vi "newRobotsLifeTime.vi"(7 "Life Time":dbl=2.0, 8 "error in (no error)":errorcluster, 9 "old robots":T1[](array[typedef]) {"height" format="%+4.3f"; "pixel_y" format="%+4.3f"; "pixel_x" format="%+4.3f"; "orientation" format="%+4.3f"; "y" format="%+4.3f"; "confidence" format="%4.3f"; "x" format="%+4.3f"}, 10 "robots":T1[](array[typedef]) {"height" format="%+4.3f"; "pixel_y" format="%+4.3f"; "pixel_x" format="%+4.3f"; "orientation" format="%+4.3f"; "y" format="%+4.3f"; "confidence" format="%4.3f"; "x" format="%+4.3f"}, 11 "Vision in":refnum<class "Vision.lvclass">) -> (0 "error out":errorcluster, 2 "robots":T1[](array[typedef]) {"height" format="%+4.3f"; "pixel_y" format="%+4.3f"; "pixel_x" format="%+4.3f"; "orientation" format="%+4.3f"; "y" format="%+4.3f"; "confidence" format="%4.3f"; "x" format="%+4.3f"}, 3 "Vision out":refnum<class "Vision.lvclass">)   [LabVIEW 2023, in "Vision.lvclass"]
uses:
  Vision.lvclass
  Old vision/Controls/SSL Detection Robot.ctl
  <vilib>/Analysis/Matrix/Datatypes/RealMatrix.ctl
  <vilib>/Analysis/NI_AALBase.lvlib
  <vilib>/Analysis/Matrix/NI_Matrix.lvlib
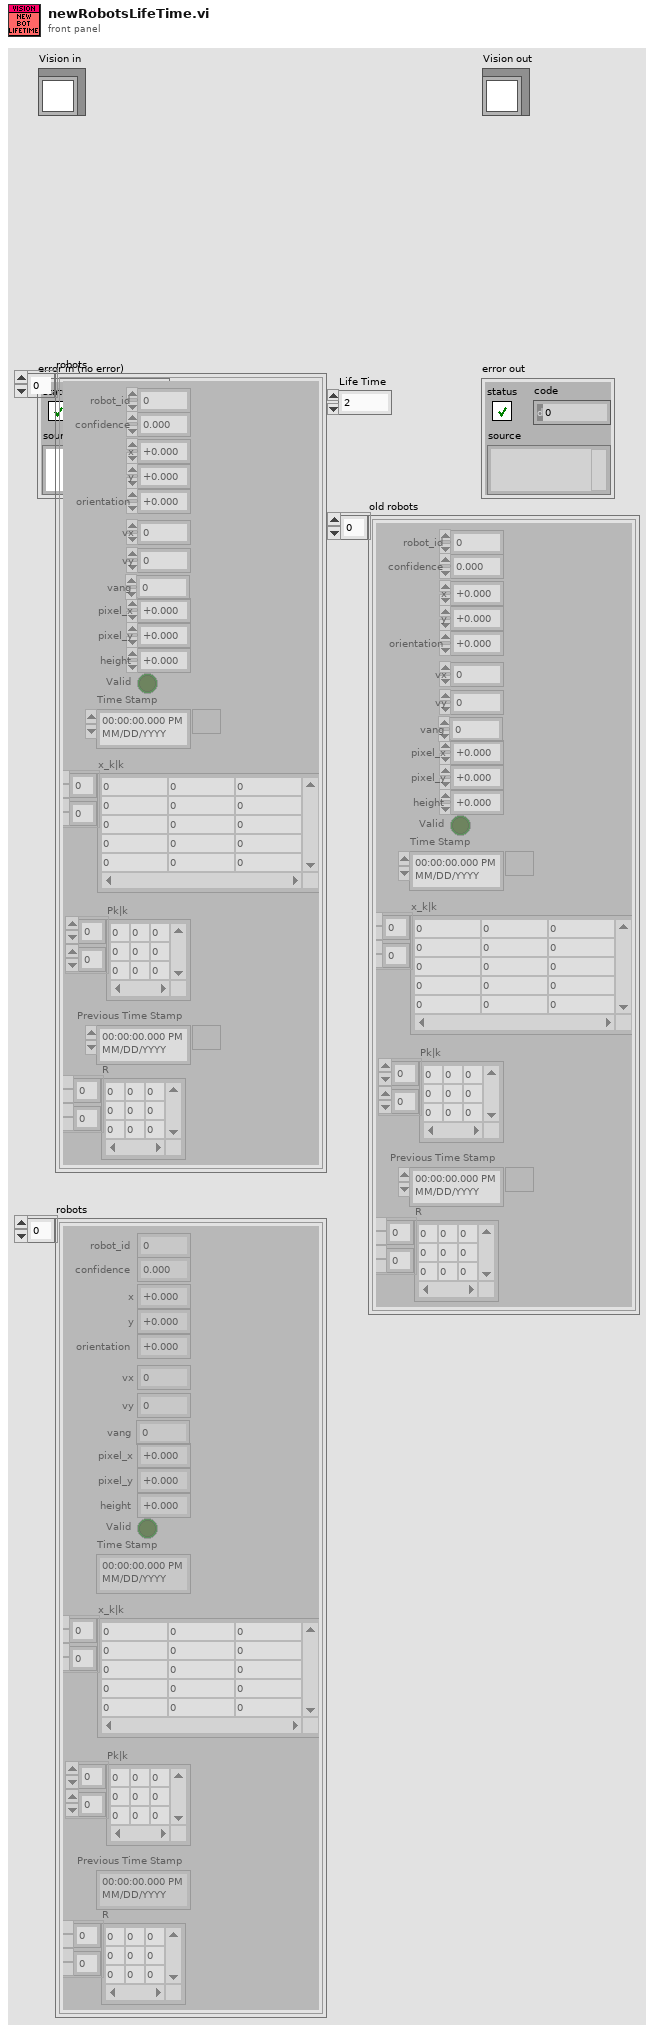
[diagram p1: front panel]
types:
  T1 = typedef "SSL Detection Robot.ctl" = cluster{"x":sgl, "robot_id":u32, "confidence":sgl, "y":sgl, "orientation":sgl, "pixel_x":sgl, "pixel_y":sgl, "height":sgl, "Valid":bool, "Time Stamp":timestamp, "x_k|k":T2, "Pk|k":T2, "Previous Time Stamp":timestamp, "R":T2, "vx":dbl, "vy":dbl, "vang":dbl}
  T2 = typedef "NI_Matrix.lvlib/RealMatrix.ctl" = dbl[][]
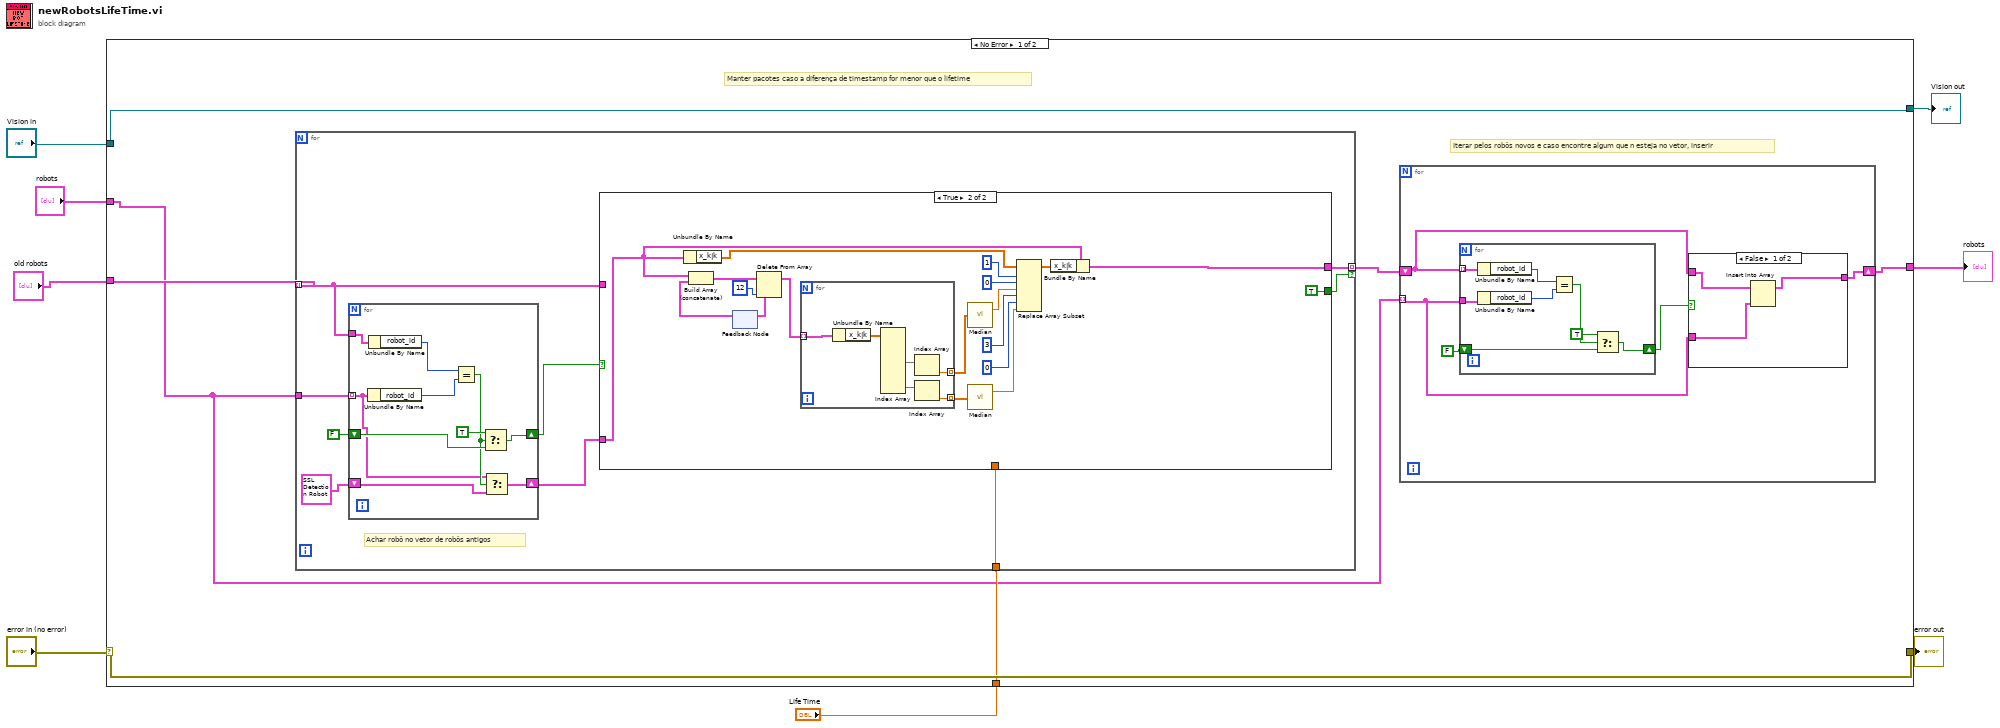
[diagram p0: block diagram]
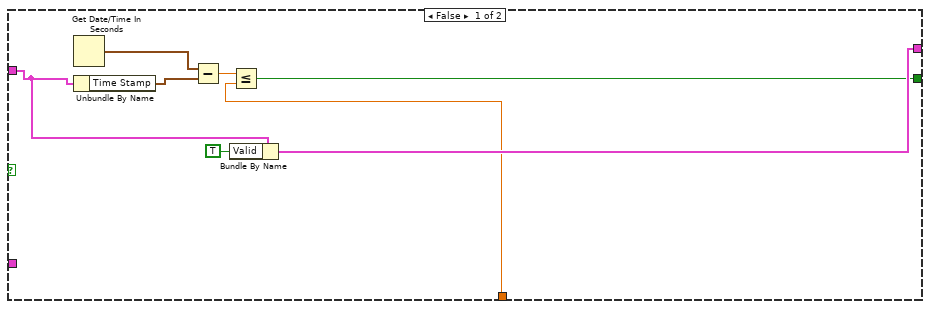
[diagram p3: hidden frame]
diagram:
  n1 = case shown="No Error" "error in (no error)" {
    selector: "error in (no error)" -> [w14 w84]
    tunnel: [w14 w84] -> w7
    tunnel: [w15 w83] -> w5
    tunnel: "Vision in" -> [w15 w83]
    tunnel: "robots" -> [w11 _]
    tunnel: "old robots" -> [w13 _]
    tunnel: "Life Time" -> [w12 _]
    tunnel: [w9 _] -> w1
    frame No Error {
      # "Iterar pelos robôs novos e caso encontre algum que n esteja no vetor, inserir"
      # "Manter pacotes caso a diferença de timestamp for menor que o lifetime"
      n2 = for {
        tunnel: w13 -> [w41] mode=indexing
        tunnel: w11 -> [w40]
        tunnel: w12 -> [w35]
        tunnel: [w34] -> w10 mode=indexing if=w33
        # "Achar robô no vetor de robôs antigos"
        n3 = for {
          tunnel: w41 -> [w51]
          tunnel: w40 -> [w44] mode=indexing
          shift-right: [w46] -> w38
          shift-left: FALSE -> [w48]
          shift-right: [w43] -> w36
          shift-left: T1 {"x"=0.0, "robot_id"=0, "confidence"=0.0, "y"=0.0, "orientation"=0.0, "pixel_x"=0.0, "pixel_y"=0.0, "height"=0.0, "Valid"=FALSE, "Time Stamp"=timestamp(0 s since 1904-01-01), "x_k|k"=[], "Pk|k"=[], "Previous Time Stamp"=timestamp(0 s since 1904-01-01), "R"=[], "vx"=0.0, "vy"=0.0, "vang"=0.0} ("Detection Robot") -> [w42]
          n4 = Unbundle By Name(w44) -> ("robot_id"=w49:u32)
          n5 = Unbundle By Name(w51) -> ("robot_id"=w50:u32)
          n6 = Equal?(x=w50, y=w49) -> (x = y?=w45:bool)
          n7 = Select(t=TRUE, s=w45, f=w48) -> (s? t:f=w46:bool)
          n8 = Select(t=w44, s=w45, f=w42) -> (s? t:f=w43:T1)
        }
        n9 = case shown="True" w38 {
          tunnel: w36 -> [_ w62]
          tunnel: [w54 w61] -> w34
          tunnel: w41 -> [w58 _]
          tunnel: w35 -> [w53 _]
          tunnel: [w52 TRUE] -> w33
          frame False {
            n10 = Get Date/Time In Seconds() -> (seconds since 1Jan1904=w59:timestamp)
            n11 = Unbundle By Name(w58) -> ("Time Stamp"=w57:timestamp)
            n12 = Subtract(x=w59, y=w57) -> (x-y=w56:dbl)
            n13 = Bundle By Name(cluster=w58, "Valid"=TRUE) -> (w54:T1)
            n14 = Less Or Equal?(x=w56, y=w53) -> (x <= y?=w52:bool)
          }
          frame True {
            n15 = Unbundle By Name(w62) -> ("x_k|k"=w70:T2)
            n16 = feedback #1() -> (w76:T1[])  [unwired: 1 in]
            n17 = Build Array (concatenate)(w62, w76) -> (w75:T1[])
            n18 = Delete From Array(array=w75, index=12) -> (array with subset deleted=w73:T1[])  [unwired: 1 in, 1 out]
            n19 = feedback-in #1(w73) -> ()
            n20 = for {
              tunnel: w73 -> [w82] mode=indexing
              tunnel: [w78] -> w72 mode=indexing
              tunnel: [w77] -> w71 mode=indexing
              n21 = Unbundle By Name(w82) -> ("x_k|k"=w81:T2)
              n22 = Index Array(array=w81) -> (element #2=w80:dbl[], element #4=w79:dbl[])  [unwired: 8 in, 2 out]
              n23 = Index Array(array=w80) -> (element=w78:dbl)  [unwired: 1 in]
              n24 = Index Array(array=w79) -> (element=w77:dbl)  [unwired: 1 in]
            }
            n25 = call <vilib>:"Median.vi"("X"=w72) -> ("median"=w67:dbl)  [unwired: 1 out]
            n26 = call <vilib>:"Median.vi"("X"=w71) -> ("median"=w64:dbl)  [unwired: 1 out]
            n27 = Replace Array Subset(array=w70, new element #1=w67, index (row) #1=1 ("index (row)"), index (col) #1=0 ("index (row)"), new element #2=w64, index (row) #2=3 ("index (row)"), index (col) #2=0 ("index (row)")) -> (w63:T2)
            n28 = Bundle By Name(cluster=w62, "x_k|k"=w63) -> (w61:T1)
          }
        }
      }
      n29 = for {
        tunnel: w11 -> [w16] mode=indexing
        shift-right: [w17] -> w9
        shift-left: w10 -> [w18]
        n30 = for {
          tunnel: w16 -> [w31]
          tunnel: w18 -> [w32] mode=indexing
          shift-right: [w25] -> w19
          shift-left: FALSE -> [w27]
          n31 = Unbundle By Name(w32) -> ("robot_id"=w30:u32)
          n32 = Unbundle By Name(w31) -> ("robot_id"=w29:u32)
          n33 = Equal?(x=w30, y=w29) -> (x = y?=w28:bool)
          n34 = Select(t=TRUE, s=w28, f=w27) -> (s? t:f=w25:bool)
        }
        n35 = case shown="False" w19 {
          tunnel: w18 -> [w23 w24]
          tunnel: [w22 w24] -> w17
          tunnel: w16 -> [w21 _]
          frame False {
            n36 = Insert Into Array(array=w23, new element=w21) -> (w22:T1[])  [unwired: 1 in]
          }
          frame True {
          }
        }
      }
    }
    frame Error {
    }
  }
  "error out" <- w7
  "Vision out" <- w5
  "robots" <- w1
